vi "Periodic Tasks.vi"(8 "error in":errorcluster) -> ()   [LabVIEW 2014]
doc: "This VI runs in parallel to other tasks. It can contain as many user-defined periodic loops as you need. These can carry out PID or other sorts of timed response."
uses:
  Robot Global Data.vi
  <vilib>/Rock Robotics/WPI/RobotDrive/WPI_RobotDriveMecanumDrive_Polar.vi
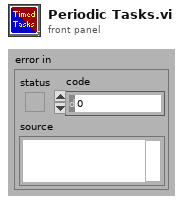
[diagram p1: front panel]
types:
  T1 = typedef "WPI_RobotDriveDevRef.ctl" = cluster{"DevStatus":errorcluster, "Motors[]":T2[], "Square Inputs":bool, "Max Output":dbl}
  T2 = typedef "WPI_MotorControlDeviceRef.ctl" = cluster{"DeviceStatus":errorcluster, "Type":T3, "PWM":cluster{"Controller":T4, "PWM Channel":T5, "DeadBand":T6}, "CAN":cluster{"Device Number":u8, "Control Mode":T7, "Semaphore":T8, "Max Vout":dbl, "TalonSRX Control Mode":T9}, "Invert":bool, "TransformRef":T10, "InvTransformRef":T10}
  T3 = typedef "WPI_MotorControlType.ctl" = enum16{"PWM", "CAN", "CANTalonSRX"}
  T4 = typedef "FPGA_TypedefDigitalModule.ctl" = enum16{"Controller 1"}
  T5 = typedef "FPGA_DIOPWMChannel.ctl" = enum8{"PWM 0", "PWM 1", "PWM 2", "PWM 3", "PWM 4", "PWM 5", "PWM 6", "PWM 7", "PWM 8", "PWM 9", "PWM MXP 0", "PWM MXP 1", "PWM MXP 2", "PWM MXP 3", "PWM MXP 4", "PWM MXP 5", "PWM MXP 6", "PWM MXP 7", "PWM MXP 8", "PWM MXP 9", "Invalid"}
  T6 = typedef "WPI_PWMDeadband.ctl" = cluster{"Name":string, "maxPositivePwm":i32, "minPositivePwm":i32, "centerPwm":i32, "maxNegativePwm":i32, "minNegativePwm":i32, "angularRange":u16}
  T7 = typedef "WPI_CANJaguar_ControlMode.ctl" = enum8{"Percent VBus", "Current", "Speed", "Position", "Voltage"}
  T8 = typedef "Semaphore RefNum" = refnum<k1>
  T9 = typedef "WPI_CANTalonSRX_APIControlMode.ctl" = enum8{"Percent VBus", "Speed", "Position", "Slave", "Unchanged / Invalid"}
  T10 = typedef "WPI_PWMTransform_ConPane.ctl" = refnum<vi>
  T11 = cluster{"Numeric":dbl, cluster{"Numeric out":dbl, "Numeric":dbl, dbl}, cluster{"Numeric":dbl, "Numeric":dbl, "upper limit":dbl, "Numeric":dbl, "Numeric":dbl, "upper limit":dbl}}
  T12 = cluster{"Numeric":dbl, "Numeric":dbl, "upper limit":dbl, "Numeric":dbl, "Numeric":dbl, "upper limit":dbl}
  T13 = cluster{cluster{"Numeric out":dbl, "Numeric":dbl, dbl}, cluster{"Numeric":dbl, "Numeric":dbl, "upper limit":dbl, "Numeric":dbl, "Numeric":dbl, "upper limit":dbl}}
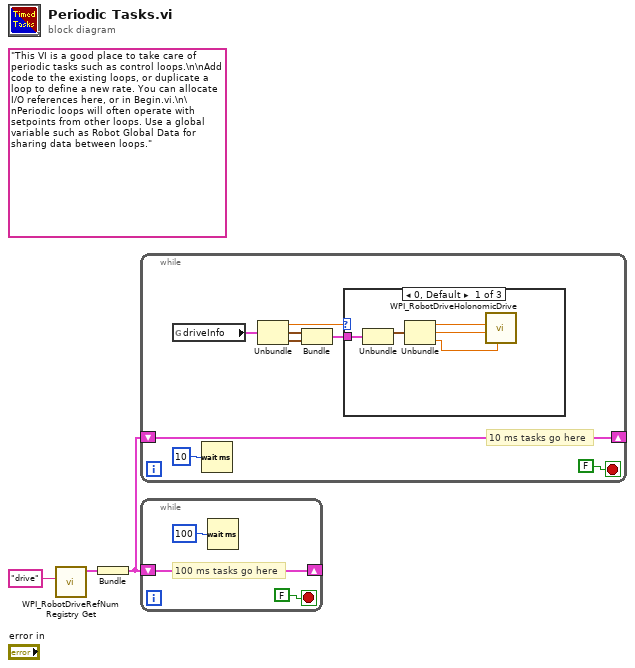
[diagram p0: block diagram]
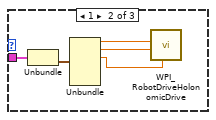
[diagram p2: hidden frame]
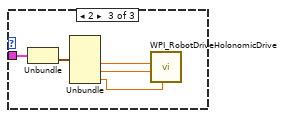
[diagram p3: hidden frame]
diagram:
  (unwired) "This VI is a good place to take care of periodic tasks such as control loops.\n\nAdd code to the existing loops, or duplicate a loop to define a new rate. You can allocate I/O references here, or in Begin.vi.\n\nPeriodic loops will often operate with setpoints from other loops. Use a global variable such as Robot Global Data for sharing data between loops."
  n1 = call <vilib>:"WPI_RobotDriveRefNum Registry Get.vi"("refnum name"="drive") -> ("RobotDriveDevRef"=w1:T1)  [unwired: 1 in, 9 out]
  n2 = Bundle("RobotDriveDevRef"=w1) -> (w2:cluster{"RobotDriveDevRef":T1})  [unwired: 1 out]
  n3 = while {
    shift-right: [w8] -> _
    shift-left: w2 -> [w8]
    stop <- FALSE stop-if-true
    # "10 ms tasks go here"
    n4 = global read "Robot Global Data.vi" "driveInfo"() -> (w9:T11)
    n5 = Wait (ms)(milliseconds to wait=u32 10) -> ()  [unwired: 1 out]
    n6 = Unbundle(w9) -> ("Numeric"=w4:dbl, w7:cluster{"Numeric out":dbl, "Numeric":dbl, dbl}, w6:T12)
    n7 = Bundle(w7, w6) -> (w5:T13)  [unwired: 1 in]
    n8 = case shown="0, Default" w4 {
      tunnel: w5 -> [w12 w17 w22]
      frame 0, Default {
        n9 = Unbundle(w12) -> (w16:cluster{"Numeric out":dbl, "Numeric":dbl, dbl})  [unwired: 1 out]
        n10 = Unbundle(w16) -> ("Numeric out"=w15:dbl, "Numeric"=w14:dbl, w13:dbl)
        n11 = call-poly <vilib>:"WPI_RobotDriveHolonomicDrive.vi"("Rotation"=w13, "Direction"=w14, "Magnitude"=w15) -> ()  [unwired: 6 in, 3 out]
      }
      frame 1 {
        n12 = Unbundle(w17) -> (w21:T12)  [unwired: 1 out]
        n13 = Unbundle(w21) -> ("Numeric"=w20:dbl, "Numeric"=w19:dbl, "upper limit"=w18:dbl)  [unwired: 3 out]
        n14 = call-poly <vilib>:"WPI_RobotDriveHolonomicDrive.vi"("Rotation"=w18, "Direction"=w19, "Magnitude"=w20) -> ()  [unwired: 6 in, 3 out]
      }
      frame 2 {
        n15 = Unbundle(w22) -> (w26:T12)  [unwired: 1 out]
        n16 = Unbundle(w26) -> ("Numeric"=w25:dbl, "Numeric"=w24:dbl, "upper limit"=w23:dbl)  [unwired: 3 out]
        n17 = call-poly <vilib>:"WPI_RobotDriveHolonomicDrive.vi"("Rotation"=w23, "Direction"=w24, "Magnitude"=w25) -> ()  [unwired: 6 in, 3 out]
      }
    }
  }
  n18 = while {
    shift-right: [w27] -> _
    shift-left: w2 -> [w27]
    stop <- FALSE stop-if-true
    # "100 ms tasks go here"
    n19 = Wait (ms)(milliseconds to wait=u32 100) -> ()  [unwired: 1 out]
  }
